vi "FFT Engine.vi"(8 "error in (no error)":errorcluster, 10 "Waveforms":waveform(dbl)[](array[waveform]), 11 "FFT config":T1 {"export mode" items=["Power Spectrum", "Power Spectral Density"]; "window" items=["Rectangle"=0, "Hanning"=1, "Hamming"=2, "Blackman-Harris"=3, "Exact Blackman"=4, "Blackman"=5, "Flat Top"=6, "4 Term B-Harris "=7, "7 Term B-Harris"=8, "Low Sidelobe"=9, "Blackman Nuttall"=11, "Triangle"=30, "Bartlett-Hanning"=31, "Bohman"=32, "Parzen"=33, "Welch"=34, "Kaiser"=60, "Dolph-Chebyshev"=61, "Gaussian"=62]; "averaging parameters"."number of averages" min=1}) -> (0 "error out":errorcluster, 1 "averaging done":bool, 2 "averages completed":dbl, 3 "Power Spectrum / PSD":cluster{"f0":dbl, "df":dbl, "magnitude":dbl[]}[](array[cluster]))   [LabVIEW 2019, in "DSP_FFT.lvclass"]
uses:
  DSP_FFT.lvclass
  <vilib>/measure/NI_MAPro.lvlib
  <vilib>/measure/maspectr.llb/FFT Power Spectrum and PSD for N Chan.vi
  <vilib>/Analysis/4window.llb/windowTd.ctl
  <vilib>/Analysis/NI_AALPro.lvlib
  <vilib>/measure/maspectr.llb/Power Spectrum and PSD Export Mode.ctl
  DSP/Typedefs/FFT_Config.ctl
  DSP/DSP.lvclass
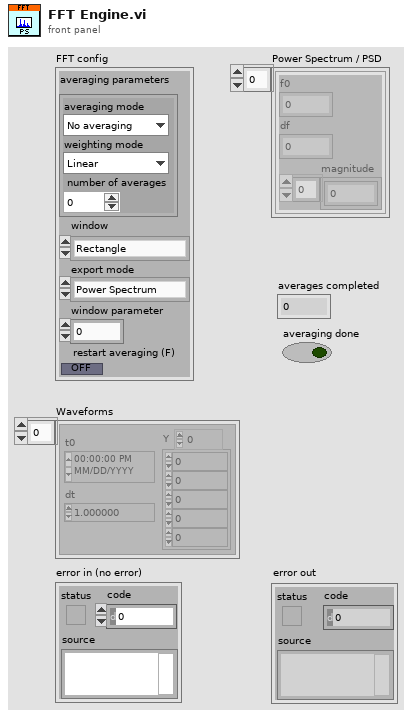
[diagram p1: front panel]
types:
  T1 = typedef "DSP.lvclass/FFT_Config.ctl" = cluster{"averaging parameters":cluster{"averaging mode":enum16{"No averaging", "Vector averaging", "RMS averaging", "Peak hold"}, "weighting mode":enum16{"Linear", "Exponential"}, "number of averages":u32}, "window":T2, "export mode":T3, "window parameter":dbl, "restart averaging (F)":bool}
  T2 = typedef "NI_AALPro.lvlib/windowTd.ctl" = u32
  T3 = typedef "NI_MAPro.lvlib/Power Spectrum and PSD Export Mode.ctl" = u16
  T4 = cluster{"averaging mode":enum16{"No averaging", "Vector averaging", "RMS averaging", "Peak hold"}, "weighting mode":enum16{"Linear", "Exponential"}, "number of averages":u32}
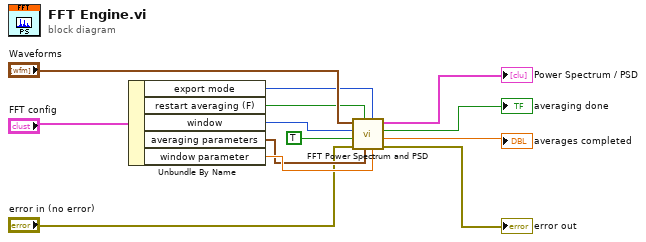
[diagram p0: block diagram]
diagram:
  n1 = Unbundle By Name("FFT config") -> ("export mode"=w8:T3, "restart averaging (F)"=w9:bool, "window"=w10:T2, "averaging parameters"=w11:T4, "window parameter"=w12:dbl)
  n2 = call-poly <vilib>:"FFT Power Spectrum and PSD.vi"("window parameter"=w12, "export mode"=w8, "averaging parameters"=w11, "restart averaging (F)"=w9, "error in (no error)"="error in (no error)", "dB On (F)"=TRUE, "window"=w10, "time signals"="Waveforms") -> ("error out"=→"error out":errorcluster, "averages completed"=→"averages completed":dbl, "averaging done"=→"averaging done":bool, "Power Spectrum / PSD"=→"Power Spectrum / PSD":cluster{"f0":dbl, "df":dbl, "magnitude":dbl[]}[])
